vi "DriveShifter.vi"(8 "error in (no error)":errorcluster, 10 "HighGear?":bool, 11 "Drive in":refnum<class "Drive.lvclass">) -> (0 "error out":errorcluster, 3 "Drive out":refnum<class "Drive.lvclass">)   [LabVIEW 2018, in "Drive.lvlib" / "Drive.lvclass"]
doc: "This VI switches the pneumatic piston from HIGH to LOW depending on the boolean that arrives. If the boolean does not change, and the switching time has elapsed, then it will keep the solenid off."
uses:
  Drive.lvclass
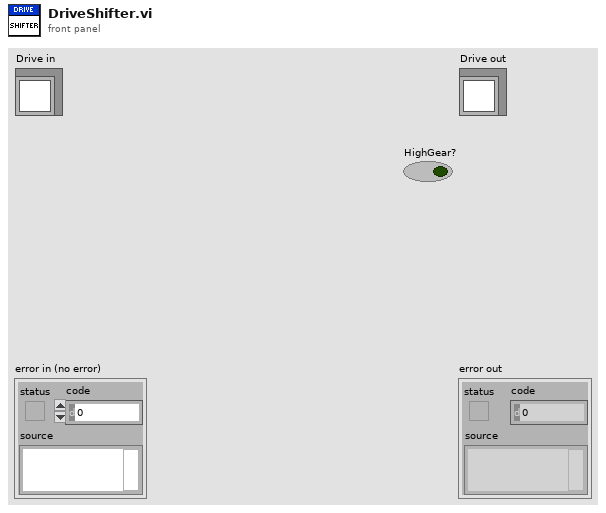
[diagram p1: front panel]
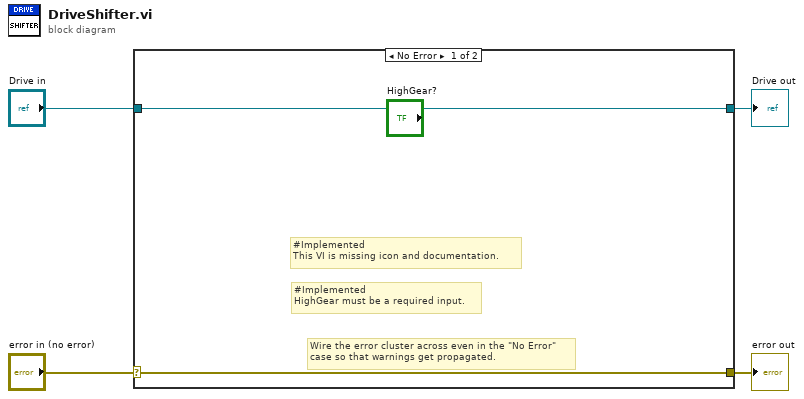
[diagram p0: block diagram]
diagram:
  n1 = case shown="No Error" "error in (no error)" {
    selector: "error in (no error)" -> [w5 w8]
    tunnel: [w5 w8] -> w3
    tunnel: [w6 w7] -> w1
    tunnel: "Drive in" -> [w6 w7]
    frame No Error {
      # "#Implemented\nHighGear must be a required input."
      # "#Implemented\nThis VI is missing icon and documentation."
      # "Wire the error cluster across even in the \"No Error\"\ncase so that warnings get propagated."
    }
    frame Error {
    }
  }
  "error out" <- w3
  "Drive out" <- w1
